vi "storeImage.vi"(8 "error in (no error)":errorcluster, 11 "ImageAnalyser in":refnum<class "ImageAnalyser.lvclass">) -> (0 "error out":errorcluster, 3 "ImageAnalyser out":refnum<class "ImageAnalyser.lvclass">)   [LabVIEW 2009, in "Tools.lvlib" / "Imaging.lvlib" / "ImageAnalyser.lvclass"]
uses:
  ImageAnalyser.lvclass
  <vilib>/vision/Image Controls.llb/IMAQ Image.ctl
panel:
  in  "Image":T1
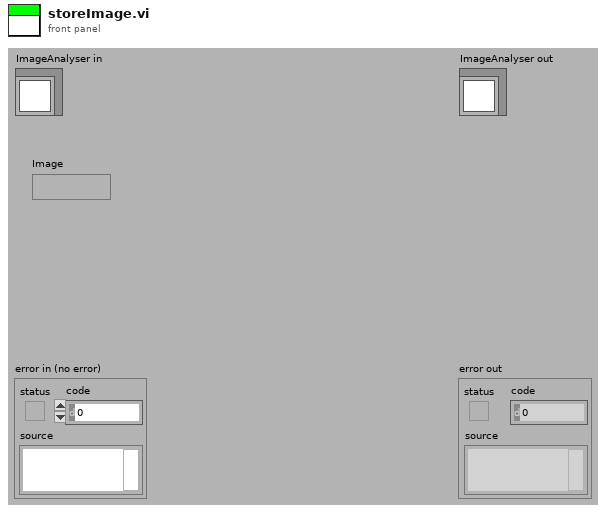
[diagram p1: front panel]
types:
  T1 = typedef "IMAQ Image.ctl" = refnum<image>
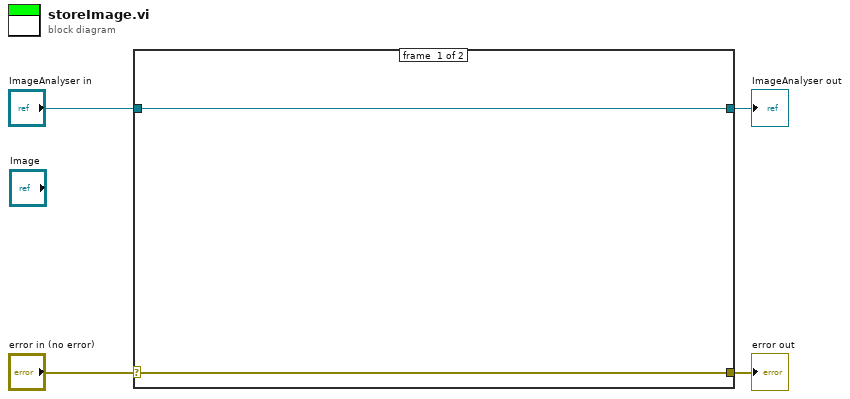
[diagram p0: block diagram]
diagram:
  n1 = case shown="No Error" "error in (no error)" {
    selector: "error in (no error)" -> [w5 w8]
    tunnel: [w5 w8] -> w3
    tunnel: [w6 w7] -> w1
    tunnel: "ImageAnalyser in" -> [w6 w7]
    frame #0 {
    }
    frame #1 {
    }
  }
  "error out" <- w3
  "ImageAnalyser out" <- w1
